vi "test-MecaDrvPoseEst2-Test1.vi"(8 "error in (no error)":errorcluster) -> (0 "error out":errorcluster, 3 "Test Passed":bool)   [LabVIEW 2019]
uses:
  <vilib>/Rock Robotics/WPI/ThirdParty/JAS_Junk/TrajLib/Rotation2d_CreateAngle.vi
  <vilib>/Rock Robotics/WPI/ThirdParty/JAS_Junk/TrajLib/MatBuilder_Create.vi
  <vilib>/Rock Robotics/WPI/ThirdParty/JAS_Junk/TrajLib/Trajectory_Library.lvlib
panel:
  out "Sub error":bool
  out "End Y pos passed":bool
  out "End X pos passed":bool
  out "AddVisionCount":i32
  out "TotalTImeSecs 2":dbl
  out "BenchProcessing \nTimer Per Pass":dbl
  out "BenchTotalTime":dbl
  out "BenchTotalPasses":dbl
  out "MaxErrPassed":bool
  out "MeanPassed":bool
  out "ErrorSumNormalized":dbl
  out "Error Sum":dbl
  out "Max Error":dbl
  out "VIsionMeasCount":i32
  out "TotalTImeSecs":dbl
  out "Position Graph":cluster{dbl[], dbl[]}[](graph)
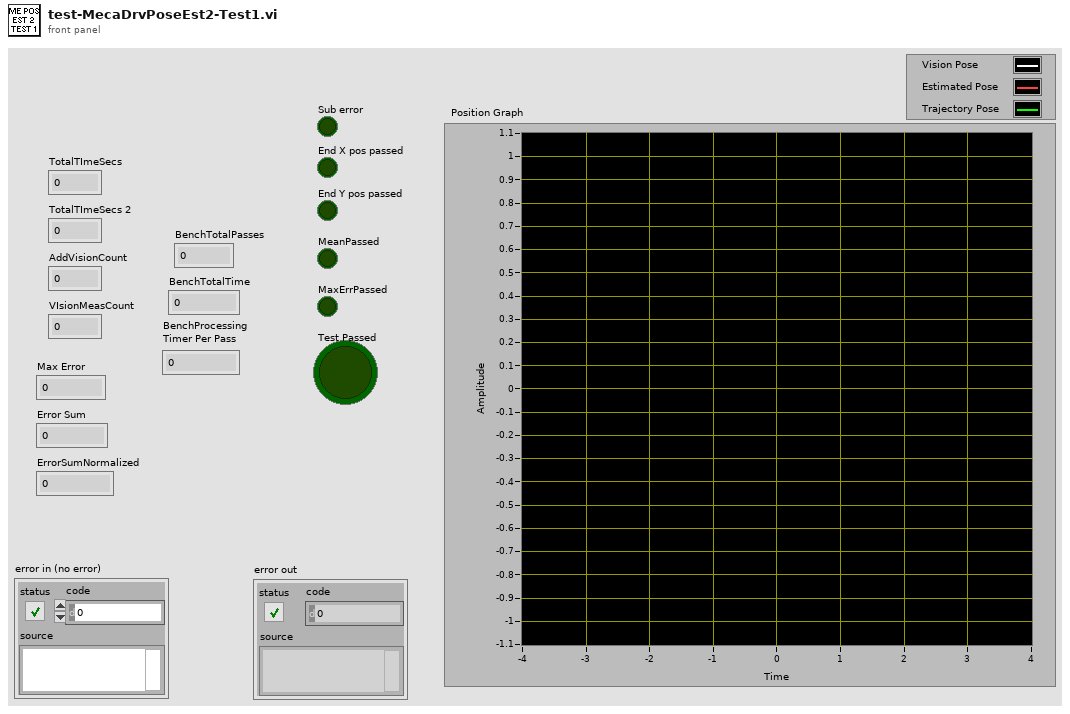
[diagram p1: front panel]
types:
  T1 = typedef "Trajectory_Library.lvlib/TRANSLATION2D.ctl" = cluster{"X":dbl, "Y":dbl}
  T2 = typedef "Trajectory_Library.lvlib/MECA_DRIVE_KINEMATICS.ctl" = cluster{"FrontLeft":T1, "FrontRight":T1, "RearLeft":T1, "RearRight":T1, "InverseKinematics":T3, "ForwardKinematics":T3, "PrevCoR":T1}
  T3 = typedef "NI_Matrix.lvlib/RealMatrix.ctl" = dbl[][]
  T4 = typedef "Trajectory_Library.lvlib/MECA_WHEEL_POSITIONS.ctl" = cluster{"FrontLeft":dbl, "FrontRight":dbl, "RearLeft":dbl, "RearRight":dbl, "P":bool}
  T5 = typedef "Trajectory_Library.lvlib/POSE2D.ctl" = cluster{"TRANSLATION":T1, "ROTATION":T6}
  T6 = typedef "Trajectory_Library.lvlib/ROTATION2D.ctl" = cluster{"VALUE":dbl, "COS":dbl, "SIN":dbl}
  T7 = typedef "Trajectory_Library.lvlib/TRAJ_CONFIG.ctl" = cluster{"MaxVelocity":dbl, "Max Acceleration":dbl, "StartVelocity":dbl, "End Velocity":dbl, "Reversed":bool, "Constraints":variant[]}
  T8 = typedef "Trajectory_Library.lvlib/MECA_DRIVE_POSE_EST2.ctl" = cluster{"M_Vision_K":T3, "m_nominal_dT":dbl, "m_PrevTime_Sec":dbl, "Pose_Buffer":T9, "Meca_Drive_Odom":T10, "M_Q":T3}
  T9 = typedef "Trajectory_Library.lvlib/TIME_INTERPOLATABLE_VARIANT.ctl" = cluster{"TimeStamps":dbl[], "DataArray":variant[], "Min_TimeStamp":dbl, "Max_TimeStamp":dbl, "ItemCount":i32, "MaxBufferTime":dbl}
  T10 = typedef "Trajectory_Library.lvlib/MECA_DRIVE_ODOMETRY.ctl" = cluster{"POSE":T5, "GyroOffset":T6, "PreviousAngle":T6, "Kinematics":T2, "PreviousWheelPositions":T4}
  T11 = typedef "Trajectory_Library.lvlib/TRAJECTORY.ctl" = cluster{"TotalTImeSecs":dbl, "States":T12[]}
  T12 = typedef "Trajectory_Library.lvlib/TRAJ_STATE.ctl" = cluster{"TimeSeconds":dbl, "Velocity":dbl, "Acceleration":dbl, "POSE":T5, "Curvature":dbl}
  T13 = cluster{"MaxErrPassed":bool, "MeanPassed":bool, "Error Sum":dbl, "ErrorSumNormalized":dbl, "Max Error":dbl, "AddVisionCount":i32, "VIsionApplyCount":i32, "BenchTotalPasses":dbl, "BenchTotalTime":dbl, "BenchProcessing \nTimer Per Pass":dbl, "TotalTImeSecs":dbl, "End X pos passed":bool, "End Y pos passed":bool, "Sub error":bool, "End X Dev":dbl, "End Y Dev":dbl}
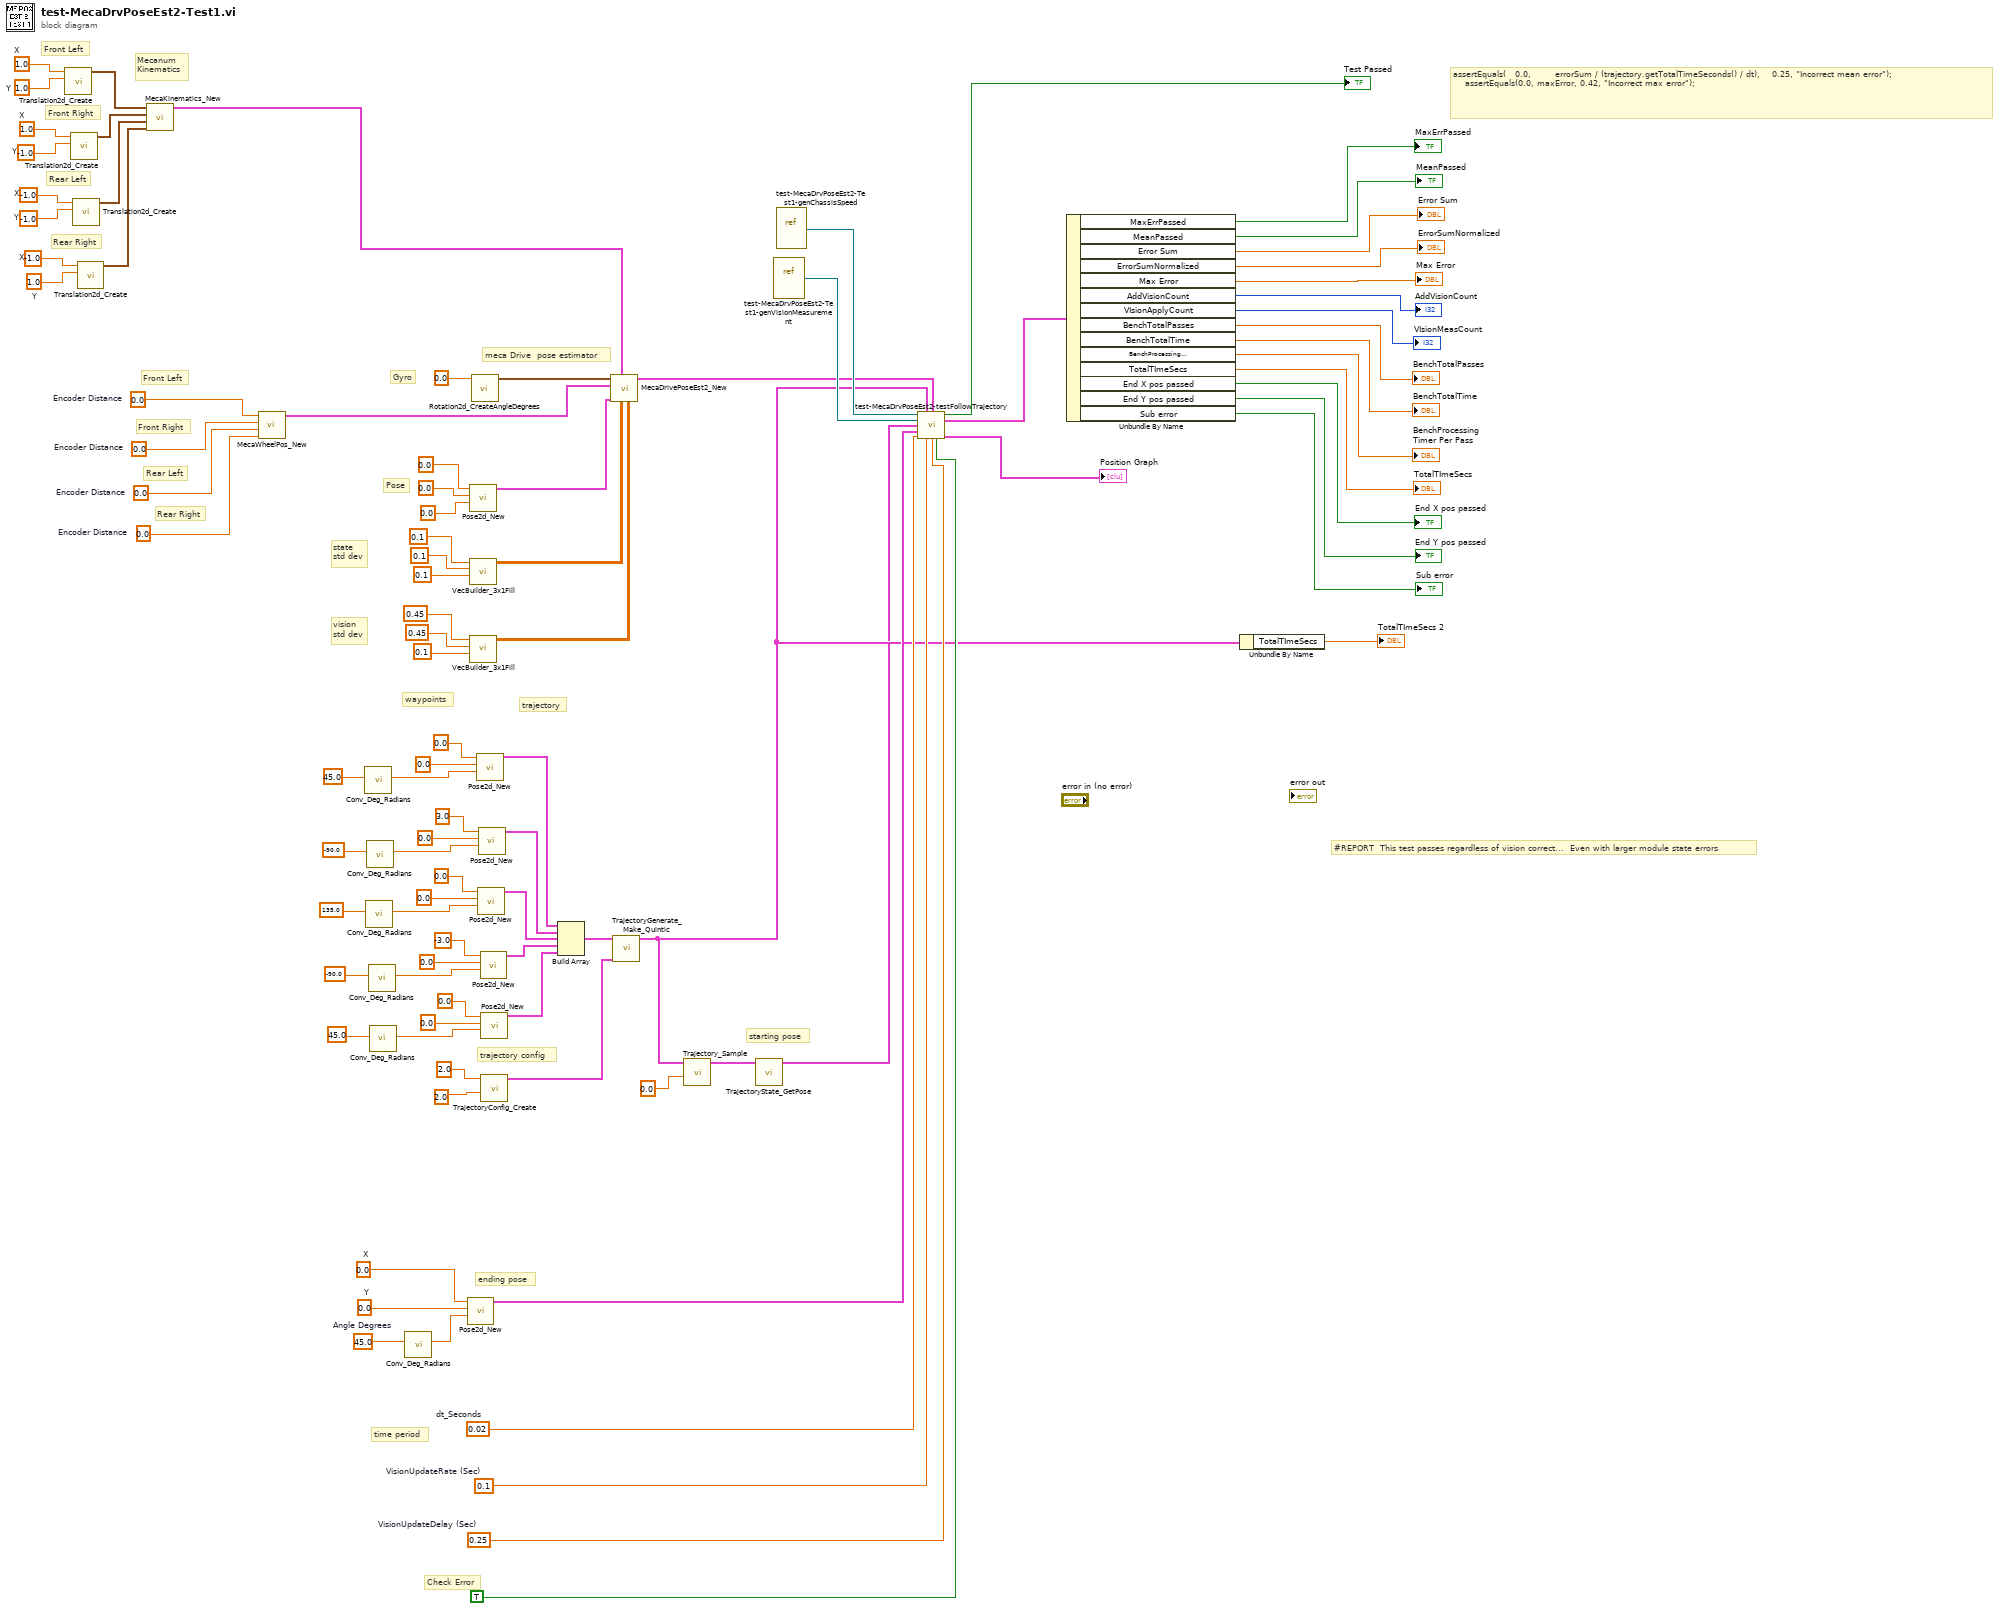
[diagram p0: block diagram]
diagram:
  w19 = -1.0  # X
  w18 = 1.0  # Y
  w17 = -1.0  # X
  w16 = -1.0  # Y
  w15 = 1.0  # X
  w14 = -1.0  # Y
  w13 = 1.0  # X
  w12 = 1.0  # Y
  w8 = 0.0  # Encoder Distance
  w9 = 0.0  # Encoder Distance
  w10 = 0.0  # Encoder Distance
  w11 = 0.0  # Encoder Distance
  w49 = 0.25  # VisionUpdateDelay (Sec)
  w50 = 0.1  # VisionUpdateRate (Sec)
  w55 = 0.0  # X
  w54 = 0.0  # Y
  w52 = 45.0  # Angle Degrees
  w56 = 0.02  # dt_Seconds
  # "Mecanum\nKinematics"
  # "Rear Right"
  # "Rear Left"
  # "Front Right"
  # "Front Left"
  # "Front Left"
  # "Rear Right"
  # "Rear Left"
  # "Front Right"
  # "starting pose"
  # "Check Error"
  # "ending pose"
  # "state \nstd dev"
  # "#REPORT  This test passes regardless of vision correct...  Even with larger module state errors"
  # "assertEquals(   0.0,        errorSum / (trajectory.getTotalTimeSeconds() / dt),    0.25, \"Incorrect mean error\");\n    assertEquals(0.0, maxError, 0.42, \"Incorrect max error\");"
  # "time period"
  # "vision \nstd dev"
  # "Pose"
  # "Gyro"
  # "meca Drive  pose estimator"
  # "trajectory config"
  # "trajectory"
  # "waypoints"
  n1 = call <vilib>:"Translation2d_Create.vi"("Y"=w12, "X"=w13) -> ("TRANSLATION"=w20:T1)  [unwired: 9 in]
  n2 = call <vilib>:"Translation2d_Create.vi"("Y"=w14, "X"=w15) -> ("TRANSLATION"=w21:T1)  [unwired: 9 in]
  n3 = call <vilib>:"Translation2d_Create.vi"("Y"=w16, "X"=w17) -> ("TRANSLATION"=w22:T1)  [unwired: 9 in]
  n4 = call <vilib>:"Translation2d_Create.vi"("Y"=w18, "X"=w19) -> ("TRANSLATION"=w23:T1)  [unwired: 9 in]
  n5 = call <vilib>:"MecaKinematics_New.vi"("RearRight"=w23, "RearLeft"=w22, "FrontRight"=w21, "FrontLeft"=w20) -> ("MECA_DRIVE_KINEMATICS"=w7:T2)  [unwired: 7 in]
  n6 = call <vilib>:"MecaWheelPos_New.vi"("RearRightPosition"=w8, "RearLeftPosition"=w9, "FrontRightPosition"=w10, "FrontLeftPosition"=w11) -> ("MECA_WHEEL_POSITIONS"=w5:T4)  [unwired: 7 in]
  n7 = call <vilib>:"Conv_Deg_Radians.vi"("Degress"=45.0 ("Heading")) -> ("Radians"=w72:dbl)  [unwired: 10 in]
  n8 = call <vilib>:"Conv_Deg_Radians.vi"("Degress"=135.0 ("Heading")) -> ("Radians"=w80:dbl)  [unwired: 10 in]
  n9 = call <vilib>:"Conv_Deg_Radians.vi"("Degress"=-90.0 ("Heading")) -> ("Radians"=w76:dbl)  [unwired: 10 in]
  n10 = call <vilib>:"Conv_Deg_Radians.vi"("Degress"=-90.0 ("Heading")) -> ("Radians"=w84:dbl)  [unwired: 10 in]
  n11 = call <vilib>:"Conv_Deg_Radians.vi"("Degress"=45.0 ("Heading")) -> ("Radians"=w88:dbl)  [unwired: 10 in]
  n12 = call <vilib>:"Conv_Deg_Radians.vi"("Degress"=w52) -> ("Radians"=w53:dbl)  [unwired: 10 in]
  n13 = call <vilib>:"Pose2d_New.vi"("Heading"=w53, "Y"=w54, "X"=w55) -> ("out POSe"=w51:T5)  [unwired: 8 in]
  n14 = call <vilib>:"Pose2d_New.vi"("Heading"=0.0, "Y"=0.0, "X"=0.0) -> ("out POSe"=w4:T5)  [unwired: 8 in]
  n15 = call <vilib>:"VecBuilder_3x1Fill.vi"("R2"=0.1 ("element"), "R1"=0.1 ("element"), "R0"=0.1 ("element")) -> ("output matrix"=w3:T3)  [unwired: 8 in]
  n16 = call <vilib>:"VecBuilder_3x1Fill.vi"("R2"=0.1 ("element"), "R1"=0.45 ("element"), "R0"=0.45 ("element")) -> ("output matrix"=w2:T3)  [unwired: 8 in]
  n17 = call <vilib>:"Rotation2d_CreateAngleDegrees.vi"("Angle_Degrees"=0.0) -> ("ROTATION"=w6:T6)  [unwired: 10 in]
  n18 = call <vilib>:"Pose2d_New.vi"("Heading"=w72, "Y"=0.0, "X"=0.0) -> ("out POSe"=w71:T5)  [unwired: 8 in]
  n19 = call <vilib>:"Pose2d_New.vi"("Heading"=w80, "Y"=0.0, "X"=0.0) -> ("out POSe"=w68:T5)  [unwired: 8 in]
  n20 = call <vilib>:"Pose2d_New.vi"("Heading"=w76, "Y"=0.0, "X"=3.0) -> ("out POSe"=w69:T5)  [unwired: 8 in]
  n21 = call <vilib>:"Pose2d_New.vi"("Heading"=w84, "Y"=0.0, "X"=-3.0) -> ("out POSe"=w67:T5)  [unwired: 8 in]
  n22 = call <vilib>:"Pose2d_New.vi"("Heading"=w88, "Y"=0.0, "X"=0.0) -> ("out POSe"=w93:T5)  [unwired: 8 in]
  n23 = call <vilib>:"TrajectoryConfig_Create.vi"("MaxAcceleration"=2.0, "MaxVelocity"=2.0) -> ("TRAJECTORY_CONFIG"=w90:T7)  [unwired: 9 in]
  n24 = Build Array(w71, w69, w68, w67, w93) -> (w91:T5[])
  n25 = call <vilib>:"MecaDrivePoseEst2_New.vi"("VisionMeasurementStdDevs"=w2, "StateStdDevs"=w3, "MECA_DRIVE_KINEMATICS"=w7, "InitialPose"=w4, "Module Positions"=w5, "gyroAngle"=w6) -> ("MecaDrivePoseEstimate"=w1:T8)  [unwired: 4 in, 1 out]
  n26 = call <vilib>:"TrajectoryGenerate_Make_Quintic.vi"("traj_config"=w90, "waypointPOSE"=w91) -> ("TRAJECTORY"=w28:T11)  [unwired: 8 in, 1 out]
  n27 = call <vilib>:"Trajectory_Sample.vi"("Time"=0.0, "InputTRAJECTORY"=w28) -> ("OutputTRAJ_STATE"=w26:T12)  [unwired: 9 in]
  n28 = call <vilib>:"TrajectoryState_GetPose.vi"("TRAJ_STATE"=w26) -> ("TrajStatePose"=w25:T5)  [unwired: 10 in]
  n29 = vi-ref "test-MecaDrvPoseEst2-Test1-genVisionMeasurement.vi"() -> (w45:refnum<vi>)
  n30 = vi-ref "test-MecaDrvPoseEst2-Test1-genChassisSpeed.vi"() -> (w46:refnum<vi>)
  n31 = call "test-MecaDrvPoseEst2-testFollowTrajectory.vi"("chassisSpeedsGenerator"=w46, "TRAJECTORY"=w28, "MecaDrivePoseEstimate2"=w1, "genVisionMeasurement"=w45, "StartingPose"=w25, "EndingPose"=w51, "dt_Seconds"=w56, "VisionUpdateRate"=w50, "VisionUpdateDelay"=w49, "CheckError"=TRUE) -> ("Test Passed"=→"Test Passed":bool, "Output Data"=w42:T13, "DataForGraph"=→"Position Graph":cluster{dbl[], dbl[]}[])  [unwired: 3 in]
  n32 = Unbundle By Name(w42) -> ("MaxErrPassed"=→"MaxErrPassed":bool, "MeanPassed"=→"MeanPassed":bool, "Error Sum"=→"Error Sum":dbl, "ErrorSumNormalized"=→"ErrorSumNormalized":dbl, "Max Error"=→"Max Error":dbl, "AddVisionCount"=→"AddVisionCount":i32, "VIsionApplyCount"=→"VIsionMeasCount":i32, "BenchTotalPasses"=→"BenchTotalPasses":dbl, "BenchTotalTime"=→"BenchTotalTime":dbl, "BenchProcessing \nTimer Per Pass"=→"BenchProcessing \nTimer Per Pass":dbl, "TotalTImeSecs"=→"TotalTImeSecs":dbl, "End X pos passed"=→"End X pos passed":bool, "End Y pos passed"=→"End Y pos passed":bool, "Sub error"=→"Sub error":bool)
  n33 = Unbundle By Name(w28) -> ("TotalTImeSecs"=→"TotalTImeSecs 2":dbl)
